vi "get reservation request info.vi"(0 "Item Ref in":T2 format="%.0x", 11 "error in (no error)":errorcluster) -> (4 "Item Ref out":T2 format="%.0x", 6 "channel type":T1, 8 "datatype":variant, 10 "Pattern":string, 15 "error out":errorcluster)   [LabVIEW 2016, in "FPGA RM System Definition API.lvlib"]
uses:
  <vilib>/NI Veristand/Custom Device API/Custom Device Item Ref.ctl
  FPGA-Resource-Manager-APIs/Source/Channel Type.ctl
  <vilib>/NI Veristand/Custom Device API/Get Item Property (Variant).vi
  <vilib>/NI Veristand/Custom Device API/Get Item Property (U16).vi
  <vilib>/NI Veristand/Custom Device API/Get Item Property (String).vi
  FPGA-Resource-Manager-APIs/Source/System Definition/FPGA RM System Definition API.lvlib
  <vilib>/NI VeriStand/Custom Device API/Custom Device API.lvlib
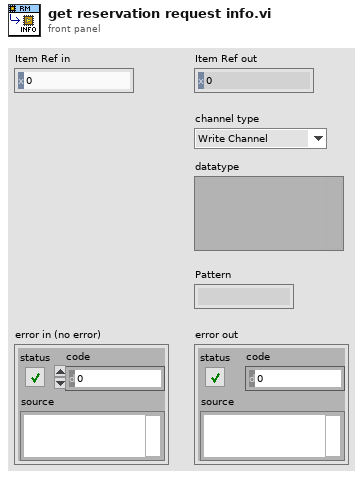
[diagram p1: front panel]
types:
  T1 = typedef "FPGA RM System Definition API.lvlib/Channel Type.ctl" = enum16{"Write Channel", "Read Channel", "Write Waveform", "Read Waveform"}
  T2 = typedef "Custom Device API.lvlib/Custom Device Item Ref.ctl" = u64
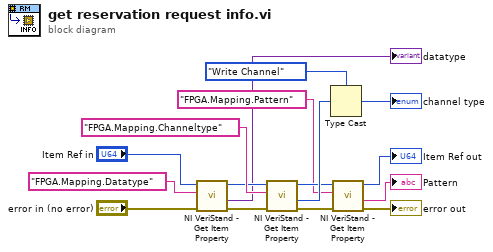
[diagram p0: block diagram]
diagram:
  n1 = call-poly <vilib>:"NI VeriStand - Get Item Property.vi"("error in (no error)"="error in (no error)", "Property Name"="FPGA.Mapping.Datatype", "Item Ref in"="Item Ref in") -> ("error out"=w15:errorcluster, "Value"=→"datatype":variant, "Item Ref out"=w12:T2)  [unwired: 5 in, 1 out]
  n2 = call-poly <vilib>:"NI VeriStand - Get Item Property.vi"("error in (no error)"=w15, "Property Name"="FPGA.Mapping.Channeltype", "Item Ref in"=w12) -> ("error out"=w16:errorcluster, "Value"=w9:u16, "Item Ref out"=w4:T2)  [unwired: 5 in, 1 out]
  n3 = Type Cast(type=Channel_Type."Write Channel" ("channel type"), x=w9) -> (*(type *) &x=→"channel type":T1)
  n4 = call-poly <vilib>:"NI VeriStand - Get Item Property.vi"("error in (no error)"=w16, "Property Name"="FPGA.Mapping.Pattern", "Item Ref in"=w4) -> ("error out"=→"error out":errorcluster, "Value"=→"Pattern":string, "Item Ref out"=→"Item Ref out":T2)  [unwired: 5 in, 1 out]
